vi "Write Format String.vi"(5 "Format String":string, 9 "NumericText in":refnum<class "NumericText.lvclass">) -> (3 "NumericText out":refnum<class "NumericText.lvclass">)   [LabVIEW 2014, in "NumericText.lvclass"]
uses:
  NumericText.lvclass
  NumericText.lvclass/NumericText.ctl
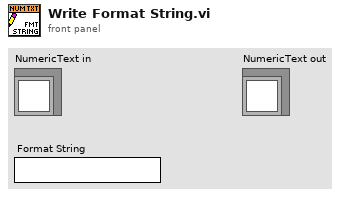
[diagram p1: front panel]
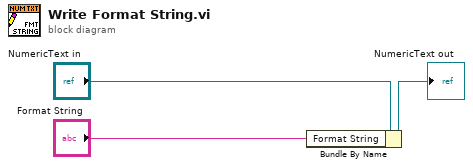
[diagram p0: block diagram]
diagram:
  n1 = Bundle By Name(cluster="NumericText in", "Format String"="Format String") -> (→"NumericText out":refnum<class "NumericText.lvclass">)
